vi "fgv_hw-info.vi"(7 "cmd":enum16{"write", "read"}(ring), 11 "HW info":T1={"AGV"=enum."ERP42", "Lidar 1"=enum."none", "Lidar 2"=enum."none", "GPS"=enum."none", "Camera"=enum."none", "Joystick"=enum."none", "sound"=enum."none"}) -> (3 "HW info out":T1={"AGV"=enum."ERP42", "Lidar 1"=enum."none", "Lidar 2"=enum."none", "GPS"=enum."none", "Camera"=enum."none", "Joystick"=enum."none", "sound"=enum."none"})   [LabVIEW 2019]
uses:
  Ctrl/system_hw.ctl
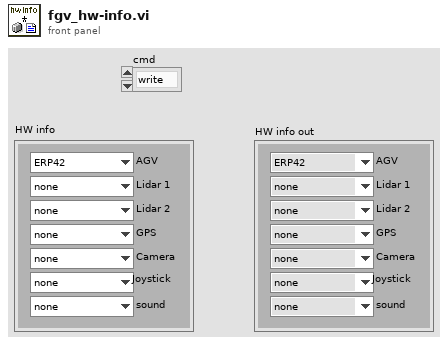
[diagram p1: front panel]
types:
  T1 = typedef "system_hw.ctl" = cluster{"AGV":enum16{"none", "ERP42", "ERP42mini", "Scout", "Ycar"}, "Lidar 1":enum16{"none", "VLP16", "TIM571", "RPLidar A2", "RPLidar A3"}, "Lidar 2":enum16{"none", "VLP16", "TIM571", "RPLidar A2", "RPLidar A3"}, "GPS":enum16{"none", "F9P", "M8P", "PwrPak7", "19X HVS"}, "Camera":enum16{"none", "C920", "C922", "GT1290C", "MS LifeCam"}, "Joystick":enum16{"none", "joystick"}, "sound":enum16{"none", "speaker"}}
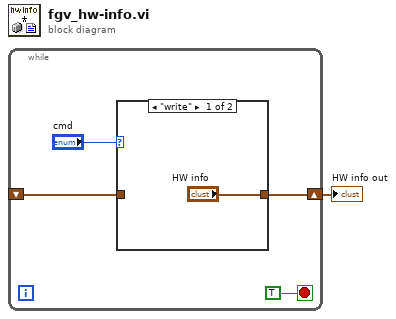
[diagram p0: block diagram]
diagram:
  n1 = while {
    shift-right: [w3] -> w1
    shift-left: _ -> [w2]
    stop <- TRUE stop-if-true
    n2 = case shown="\"write\"" "cmd" {
      tunnel: ["HW info" w7] -> w3
      tunnel: w2 -> [_ w7]
      frame "write" {
      }
      frame "read", Default {
      }
    }
  }
  "HW info out" <- w1
